vi "Create Transfers.vi"(5 "Group String Buffer":refnum<class "Buffer.lvclass">, 7 "Group Async Buffer":refnum<class "DBL Pointer.lvclass">, 8 "error in (no error)":errorcluster, 9 "starting id":i32, 10 "Transfer Configurations":T1[](array[typedef]) {"channels"."dst buffer offset" format="%d bytes"; "channels"."src buffer offset" format="%d bytes"}, 11 "Framework in":refnum<class "Framework.lvclass">) -> (0 "error out":errorcluster, 1 "ending id":i32, 2 "Transfers":refnum<class "Transfer.lvclass">[](array[class]), 3 "Framework out":refnum<class "Framework.lvclass">)   [LabVIEW 2017, in "DSF Core.lvlib" / "Framework.lvclass"]
uses:
  Framework.lvclass
  Transfer/Transfer.lvclass
  DSF Configuration API/Public/Controls/DSF Engine Transfer Configuration.ctl
  DSF Configuration API/Public/Controls/DSF Byte Order.ctl
  DSF Configuration API/Public/Controls/DSF Engine Channel Configuration.ctl
  DSF Configuration API/Public/Controls/DSF Data Type.ctl
  DSF Configuration API/Public/Controls/DSF Settings Info.ctl
  Buffer/Buffer.lvclass
  C:/Program Files (x86)/National Instruments/LabVIEW 2017/vi.lib/NI/Memory Manager/Classes/Pointer/Memory.Pointer.lvclass
  Pointer/DBL Pointer.lvclass
  <vilib>/NI/Memory Manager/Classes/Pointer/Memory.Pointer.lvclass/Memory.Pointer.ctl
  Shared/VIs/Sizeof.vi
  <vilib>/NI/Memory Manager/Classes/Pointer/Memory.Pointer.Parameter Check.Subset.vi
  <vilib>/NI/Memory Manager/Classes/Pointer/Memory.Pointer.Get Address.vi
  <vilib>/NI/Memory Manager/Classes/Pointer/Memory.Pointer.Encapsulate.vi
  <vilib>/NI/Memory Manager/Classes/Pointer/Memory.Pointer.Parameter Check.Null Pointer.vi
  <vilib>/NI/Memory Manager/Classes/Pointer/Memory.Pointer.Errors.vi
  <vilib>/NI/Memory Manager/Classes/Pointer/Memory.Pointer.Errors.Out of Bounds.vi
  <vilib>/NI/Memory Manager/Classes/Pointer/Memory.Pointer.Get Size.vi
  <vilib>/NI/Memory Manager/Classes/Pointer/Memory.Pointer.Set Size.vi
  <vilib>/NI/Memory Manager/Classes/Pointer/Memory.Pointer.Set Address.vi
  <vilib>/NI/Memory Manager/Classes/Pointer/Memory.Pointer.Set Allocated.vi
  <vilib>/NI/Memory Manager/Classes/Pointer/Memory.Pointer.Errors.Null Pointer.vi
  <vilib>/NI/Memory Manager/VIs/Source.Write.String.vi
  <vilib>/NI/Memory Manager/Classes/Pointer/Memory.Pointer.Errors.Write Pointer Size.vi
  <vilib>/NI/Memory Manager/Classes/Pointer/Memory.Pointer.Errors.Create Error.vi
  <vilib>/NI/Memory Manager/VIs/Source.Write.Scalar.Base10.vi
  <vilib>/NI/Memory Manager/VIs/Source.Write.Scalar.Base10 (U64).vi
  <vilib>/NI/Memory Manager/VIs/New Error Cluster Constant.vi
  <vilib>/NI/Memory Manager/VIs/New Error Cluster Constant (512B).vi
  <vilib>/NI/Memory Manager/VIs/Error Cluster.Set Status.vi
  <vilib>/NI/Memory Manager/VIs/Error Cluster.Set Code.vi
  <vilib>/NI/Memory Manager/VIs/Error Cluster.Set VI Source.vi
  <vilib>/NI/Memory Manager/Constants/Memory.Constants.vi
  <vilib>/NI/Memory Manager/Constants/Memory.Constants.Library Name.vi
  <vilib>/NI/Memory Manager/Classes/Pointer/Memory.Pointer.Errors.Get Info.vi
  DSF Core.lvlib
  <vilib>/NI/Memory Manager/Classes/Pointer/Memory.Pointer.lvclass
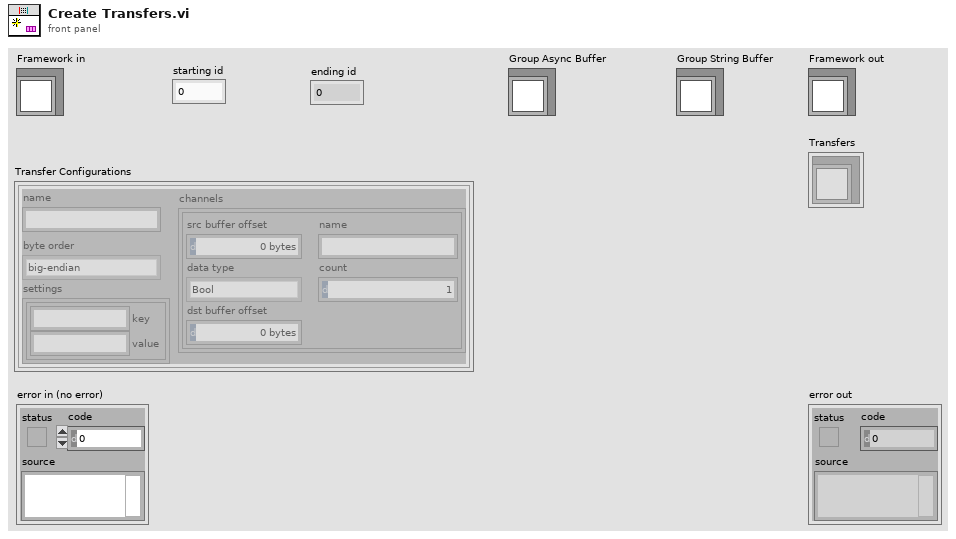
[diagram p1: front panel]
types:
  T1 = typedef "DSF Core.lvlib/DSF Engine Transfer Configuration.ctl" = cluster{"name":string, "byte order":T2, "channels":T3[], "settings":T5}
  T2 = typedef "DSF Core.lvlib/DSF Byte Order.ctl" = enum8{"big-endian", "little-endian"}
  T3 = typedef "DSF Core.lvlib/DSF Engine Channel Configuration.ctl" = cluster{"src buffer offset":u64, "name":string, "data type":T4, "count":u64, "dst buffer offset":u64}
  T4 = typedef "DSF Core.lvlib/DSF Data Type.ctl" = enum8{"Bool", "SGL", "DBL", "I8", "I16", "I32", "I64", "U8", "U16", "U32", "U64"}
  T5 = typedef "DSF Core.lvlib/DSF Settings Info.ctl" = cluster{"key":string, "value":string}[]
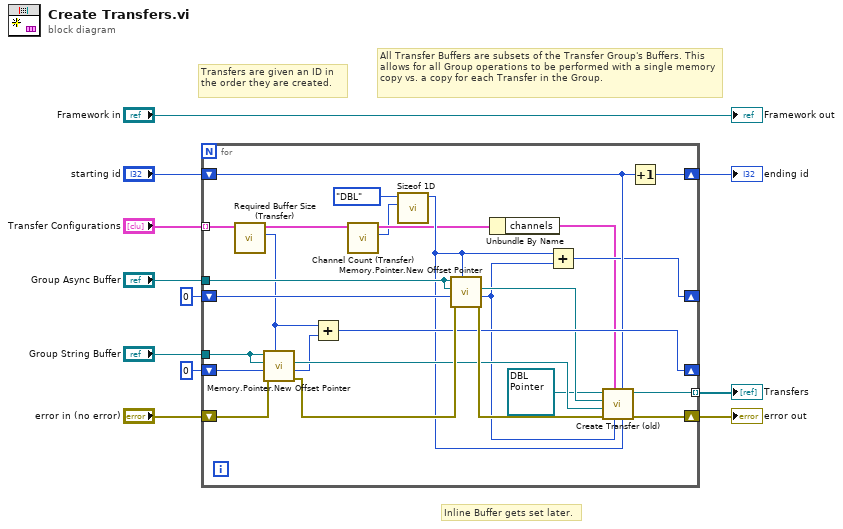
[diagram p0: block diagram]
diagram:
  # "Inline Buffer gets set later."
  # "All Transfer Buffers are subsets of the Transfer Group's Buffers. This allows for all Group operations to be performed with a single memory copy vs. a copy for each Transfer in the Group."
  # "Transfers are given an ID in the order they are created."
  n1 = for {
    shift-right: [w35] -> w11
    shift-left: "error in (no error)" -> [w27]
    tunnel: [w34] -> w1 mode=indexing
    tunnel: "Transfer Configurations" -> [w32] mode=indexing
    tunnel: "Group Async Buffer" -> [w21]
    shift-right: [w22] -> _
    shift-left: u64 0 -> [w19]
    tunnel: "Group String Buffer" -> [w25]
    shift-right: [w28] -> _
    shift-left: u64 0 -> [w30]
    shift-right: [w24] -> w3
    shift-left: "starting id" -> [w23]
    n2 = call "Required Buffer Size (Transfer).vi"("Transfer Configuration in"=w32) -> ("required buffer size"=w12:u64, "Transfer Configuration out"=w31:T1)  [unwired: 8 in, 1 out]
    n3 = call <vilib>:"Memory.Pointer.New Offset Pointer.vi"("length (-1: rest)"=w12, "error in (no error)"=w27, "offset (0)"=w30, "offset Pointer type"=w25, "base Pointer in"=w25) -> ("error out"=w37:errorcluster, "offset out"=w26:u64, "offset Pointer"=w29:refnum<class "Buffer.lvclass">)  [unwired: 3 in, 1 out]
    n4 = Add(x=w12, y=w26) -> (x+y=w28:u64)
    n5 = call "Channel Count (Transfer).vi"("Transfer Configuration in"=w31) -> ("total channel count"=w13:u64, "Transfer Configuration out"=w15:T1)  [unwired: 8 in, 1 out]
    n6 = call "Sizeof 1D.vi"("count"=w13, "data type"=DSF_Data_Type."DBL") -> ("size in bytes"=w16:u64)  [unwired: 9 in]
    n7 = call <vilib>:"Memory.Pointer.New Offset Pointer.vi"("length (-1: rest)"=w16, "error in (no error)"=w37, "offset (0)"=w19, "offset Pointer type"=w21, "base Pointer in"=w21) -> ("error out"=w36:errorcluster, "offset out"=w17:u64, "offset Pointer"=w20:refnum<class "DBL Pointer.lvclass">)  [unwired: 3 in, 1 out]
    n8 = Unbundle By Name(w15) -> ("channels"=w14:T3[])
    n9 = Add(x=w16, y=w17) -> (x+y=w22:u64)
    n10 = call "Create Transfer (old).vi"("size"=w16, "id"=w23, "group offset"=w17, "channel blocks"=w14, "error in (no error)"=w36, "String Buffer"=w29, "Intermediate Buffer"=w20, "Inline Buffer"=refnum<class "DBL Pointer.lvclass"> refnum) -> ("error out"=w35:errorcluster, "Transfer out"=w34:refnum<class "Transfer.lvclass">)  [unwired: 2 in]
    n11 = Increment(x=w23) -> (x+1=w24:i32)
  }
  "error out" <- w11
  "Transfers" <- w1
  "ending id" <- w3
  "Framework out" <- "Framework in"
